vi "首页.vi"() -> ()   [LabVIEW 2016]
uses:
  <vilib>/Utility/miscctls.llb/LVPointTypeDef.ctl
  <vilib>/Utility/sysdir.llb/System Directory Type.ctl
  <vilib>/addons/database/_DB Variant To Data/Database Variant To Data.xnode
  PLC/PLC.lvlib
panel:
  out "大项目框 12":T1(xcontrol)
  out "大项目框 11":T1(xcontrol)
  out "大项目框 10":T1(xcontrol)
  out "大项目框 9":T1(xcontrol)
  out "大项目框 8":T1(xcontrol)
  out "大项目框 7":T1(xcontrol)
  out "大项目框 6":T1(xcontrol)
  out "大项目框 5":T1(xcontrol)
  out "大项目框 4":T1(xcontrol)
  out "大项目框 3":T1(xcontrol)
  out "大项目框 2":T1(xcontrol)
  out "大项目框":T1(xcontrol)
  out "湿度":string="75.5 %"
  out "室温":string="25.8 ℃"
  # "室温:"
  # "湿度:"
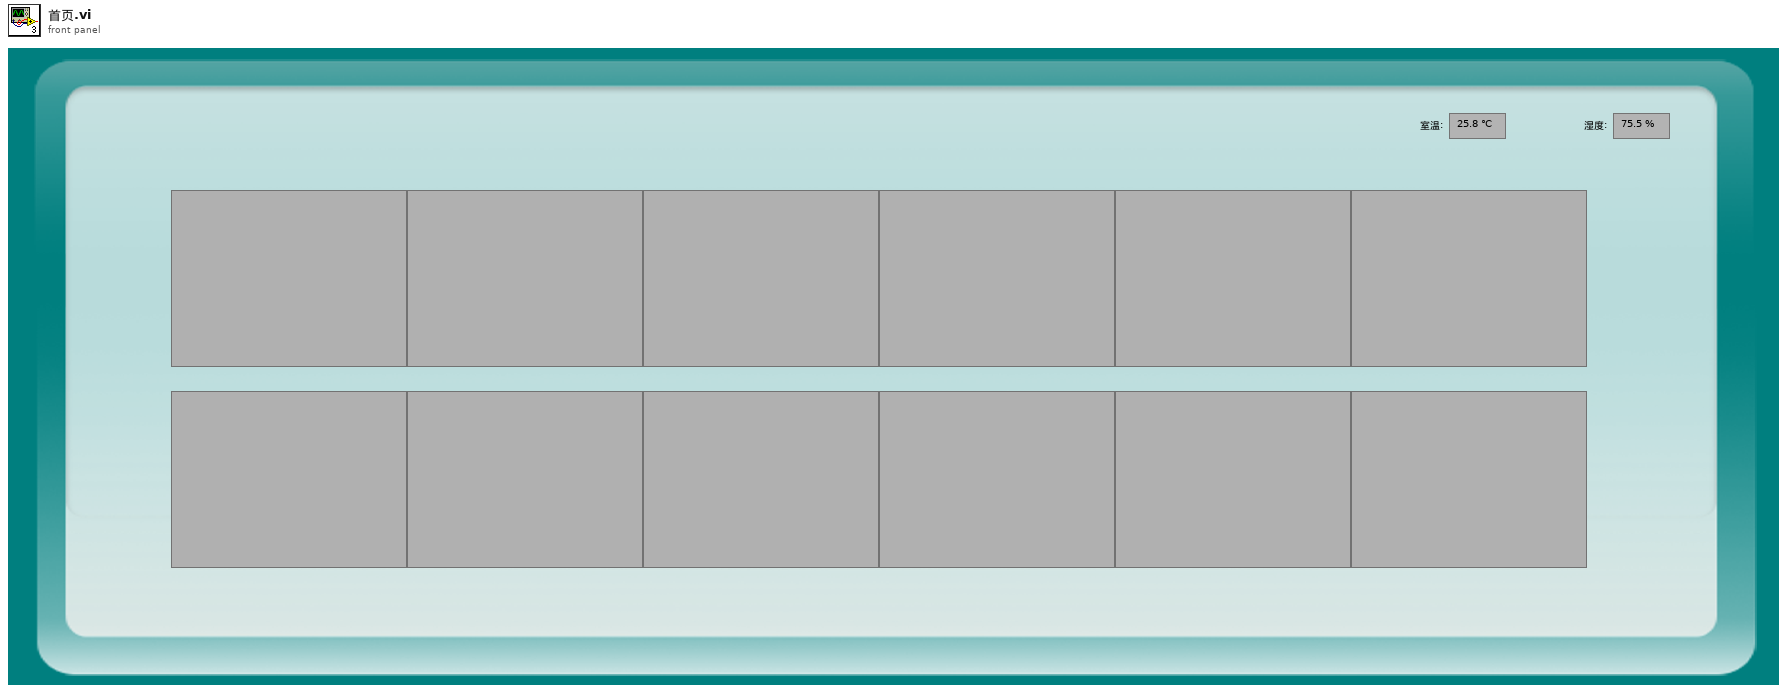
[diagram p1: front panel]
types:
  T1 = cluster{"中文项目名称":string, "英文项目名称":string, "单位":string, "浓度值":string}
  T2 = typedef "LVPointTypeDef.ctl" = cluster{"Horizontal":i16, "Vertical":i16}
  T3 = cluster{"显示参数中文名":string, "显示参数英文名":string, "显示浓度":string, "显示单位":string}[]
  T4 = cluster{"显示参数中文名":string, "显示参数英文名":string, "显示浓度":string, "显示单位":string}
  T5 = typedef "System Directory Type.ctl" = i32
  T6 = cluster{"水温":bool, "pH":bool, "DO":bool, "Cond":bool, "Turb":bool, "氨氮":bool, "总磷":bool, "总氮":bool, "CODMn":bool, "CODCr":bool, "水位":bool, "流速":bool, "瞬时流量":bool, "室温":bool, "湿度":bool}
  T7 = cluster{"AD0":sgl, "AD1":sgl, "AD2":sgl, "AD3":sgl, "AD4":sgl, "AD5":sgl}
  T8 = typedef "LVDateTimeRec.ctl" = cluster{"秒数的小数部分":dbl, "秒":i32, "分":i32, "时":i32, "日":i32, "月":i32, "年":i32, "天数（周）":i32, "天数（年）":i32, "DST":i32}
  T9 = cluster{"时间标识":timestamp, "监测值":sgl, "单位":string}
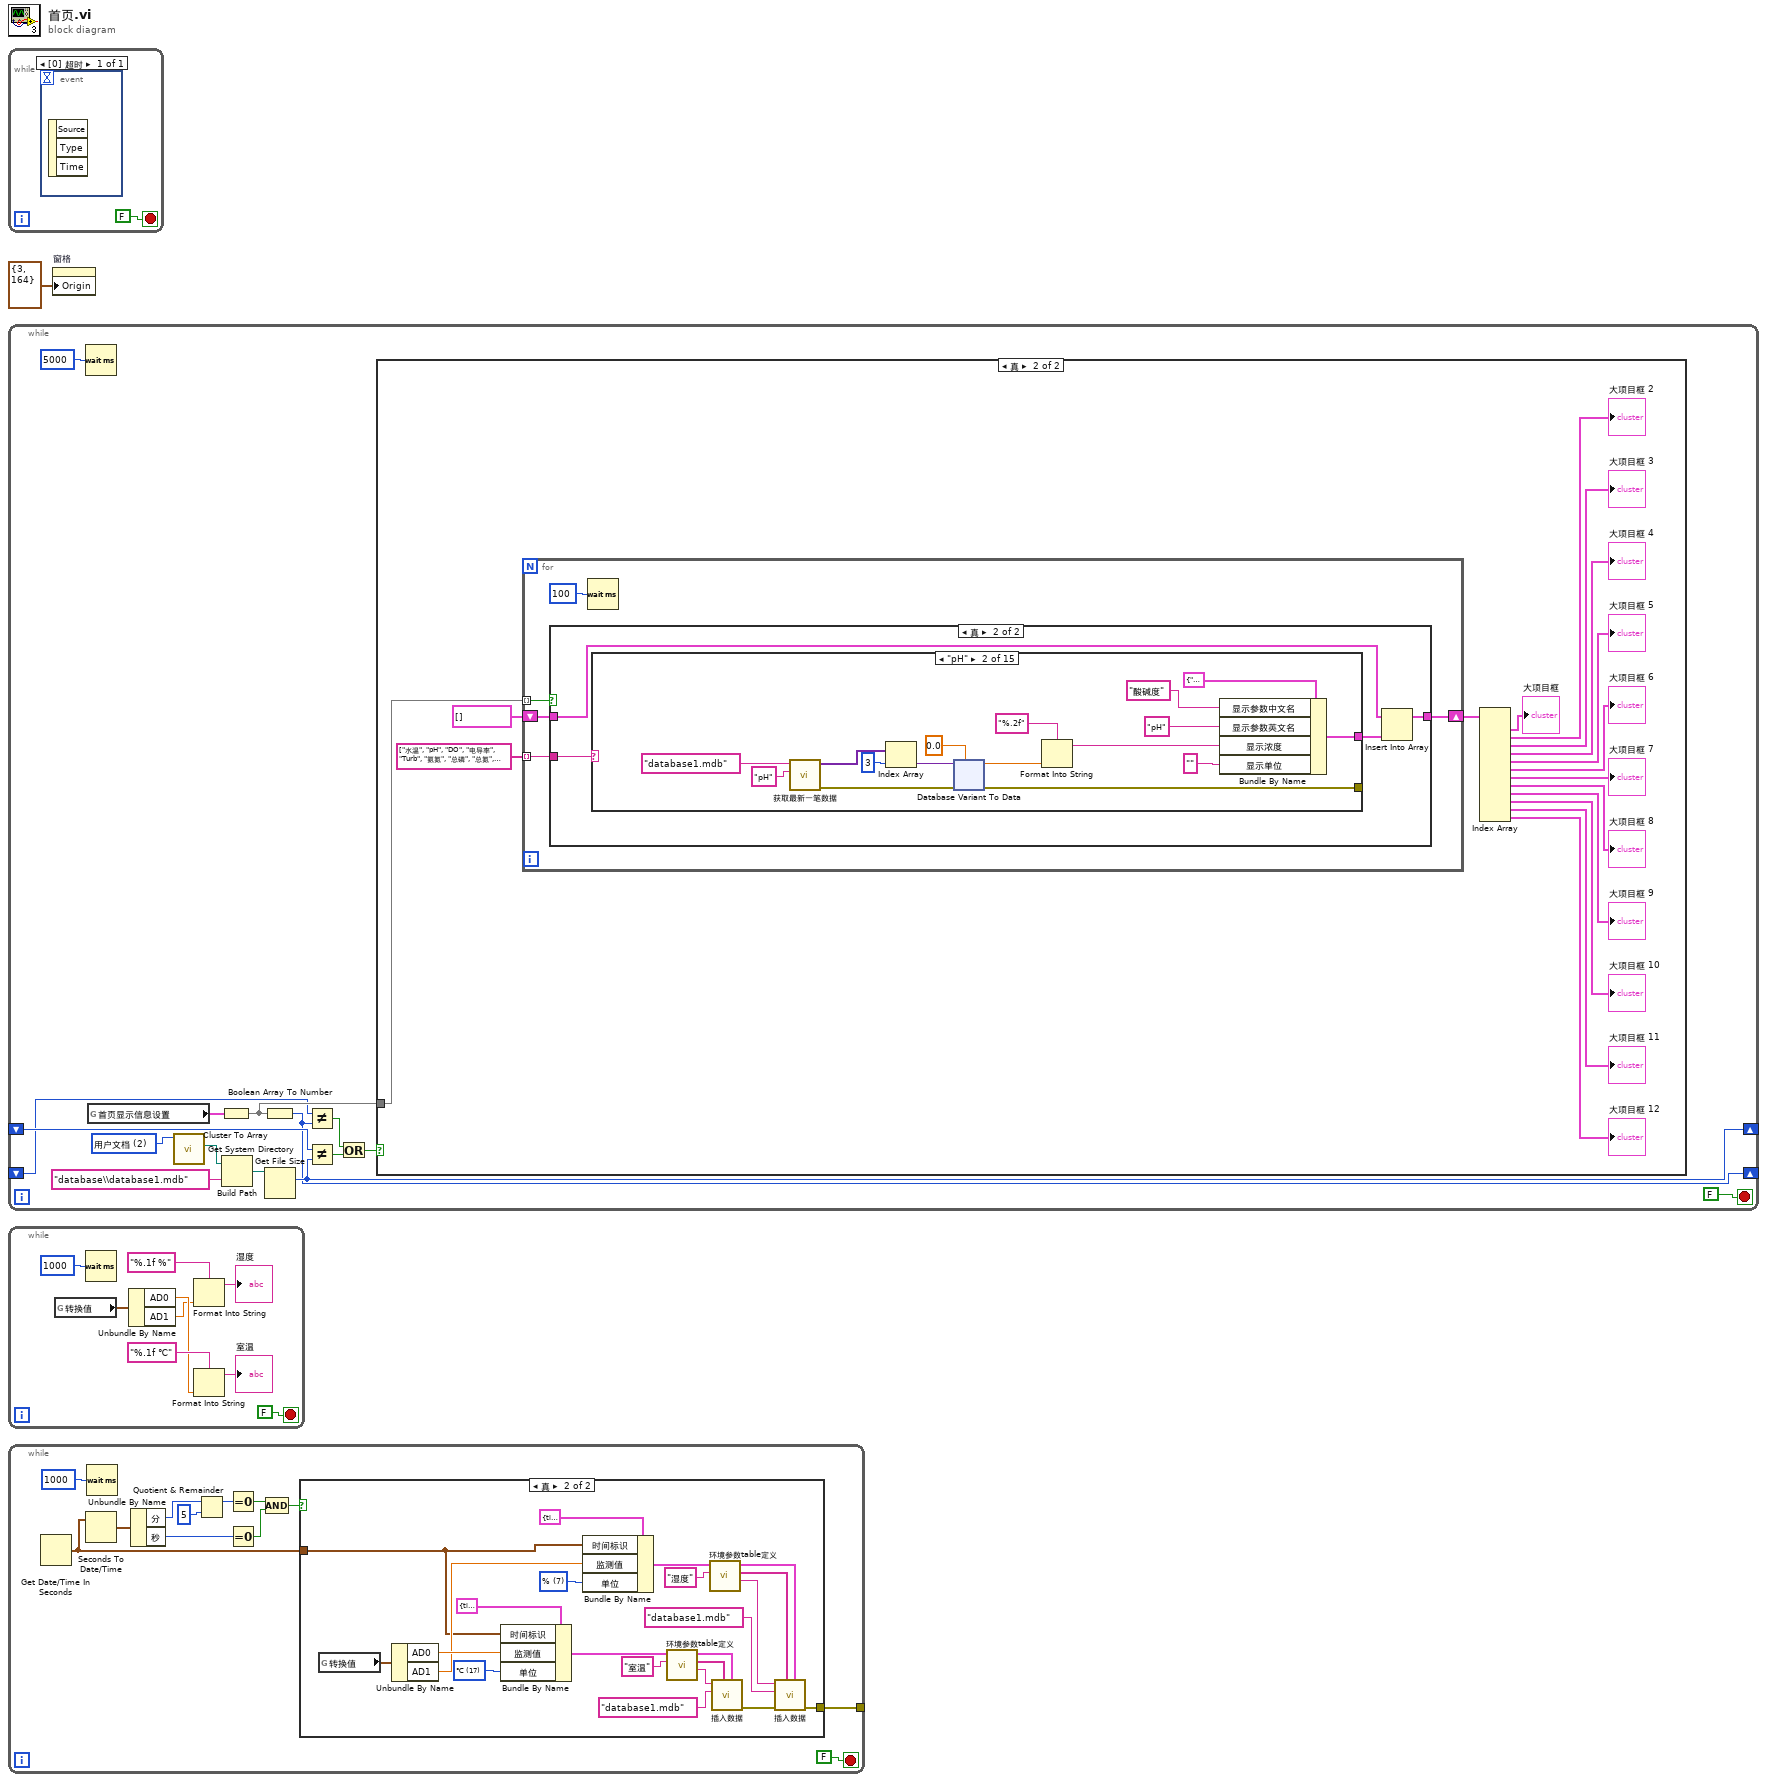
[diagram p0: block diagram]
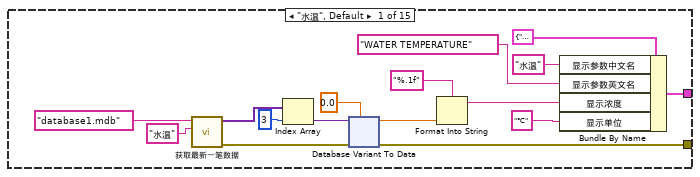
[diagram p5: hidden frame]
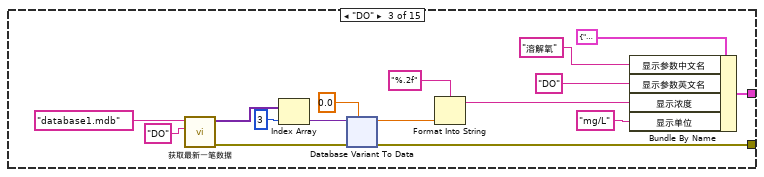
[diagram p6: hidden frame]
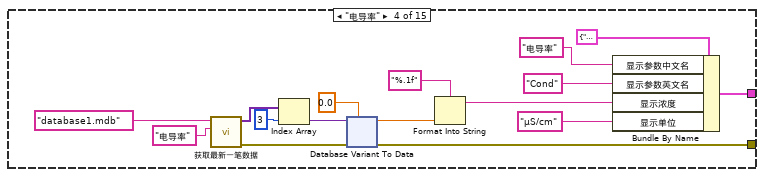
[diagram p7: hidden frame]
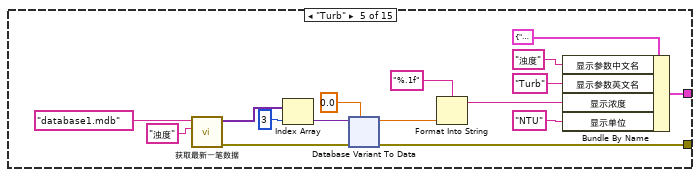
[diagram p8: hidden frame]
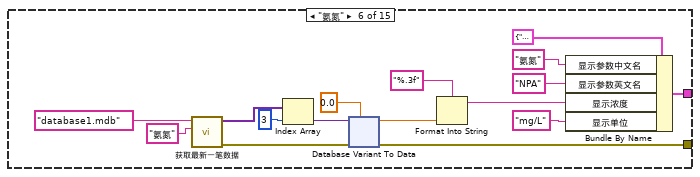
[diagram p9: hidden frame]
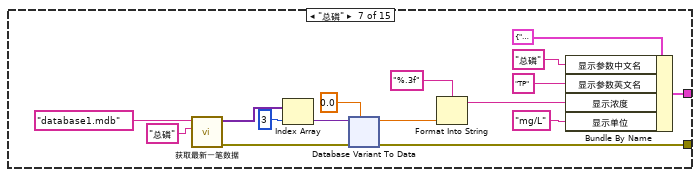
[diagram p10: hidden frame]
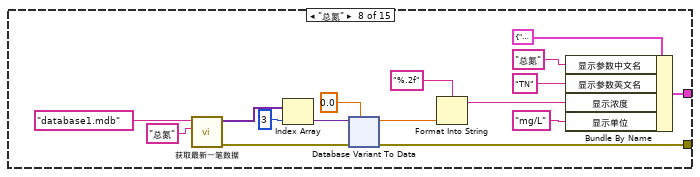
[diagram p11: hidden frame]
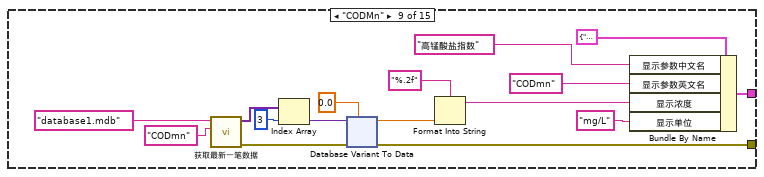
[diagram p12: hidden frame]
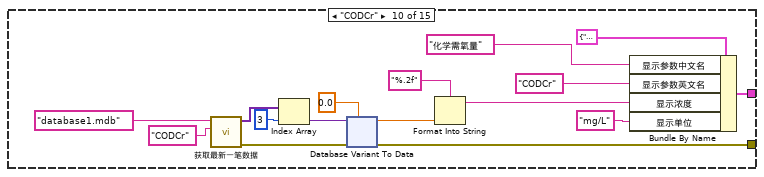
[diagram p13: hidden frame]
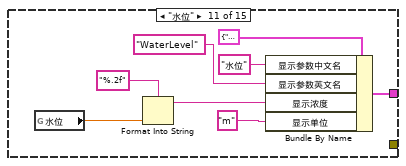
[diagram p14: hidden frame]
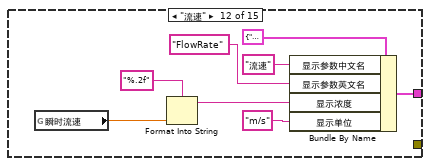
[diagram p15: hidden frame]
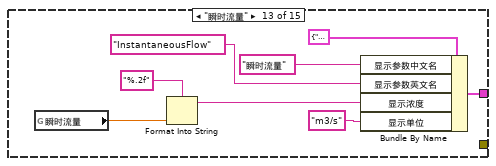
[diagram p16: hidden frame]
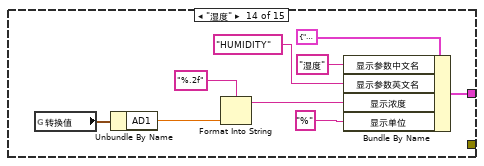
[diagram p17: hidden frame]
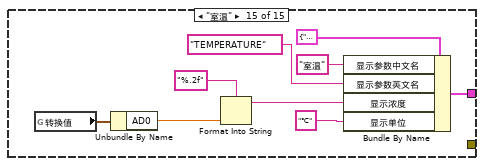
[diagram p18: hidden frame]
diagram:
  n1 = while {
    stop <- FALSE stop-if-true
    n2 = event shown="[0] 超时" {
      selector: _ -> [_]
      dyn-events: _ -> [_]
      timeout: _ -> [_]
      event Timeout {
        n3 = event-data() -> ()  [unwired: 1 in, 3 out]
      }
    }
  }
  n4 = while {
    shift-right: [w9] -> _
    shift-left: _ -> [w10]
    shift-right: [w7] -> _
    shift-left: _ -> [w6]
    stop <- FALSE stop-if-true
    w14 = T5 2 items=["用户目录"=0, "用户桌面"=1, "用户文档"=2, "用户应用程序数据"=3, "用户设置"=4, "用户临时目录"=5, "公共文档"=6, "公共应用程序数据"=7, "公共设置"=8, "公共缓存"=13, "系统核心库"=9, "系统安装库"=10, "应用程序文件"=11, "启动盘根目录"=12] ("system directory type")
    n5 = Wait (ms)(milliseconds to wait=u32 5000 ("等待时间（毫秒）")) -> ()  [unwired: 1 out]
    n6 = global read "系统设置全局变量.vi" "首页显示信息设置"() -> (w15:T6)
    n7 = call <vilib>:"Get System Directory.vi"("system directory type"=w14) -> ("system directory"=w13:path)  [unwired: 10 in]
    n8 = Cluster To Array(cluster=w15) -> (array=w8:bool[])
    n9 = Build Path(base path=w13, name or relative path="database\\database1.mdb" ("名称或相对路径")) -> (appended path=w11:path)
    n10 = Boolean Array To Number(Boolean array=w8) -> (number=w7:u32)
    n11 = Get File Size(file=w11) -> (size (in bytes)=w9:i64)  [unwired: 1 in, 2 out]
    n12 = Not Equal?(x=w6, y=w7) -> (x != y?=w4:bool)
    n13 = Not Equal?(x=w10, y=w9) -> (x != y?=w5:bool)
    n14 = Or(x=w4, y=w5) -> (x .or. y?=w3:bool)
    n15 = case shown="真" w3 {
      tunnel: w8 -> [_ w18]
      frame False {
      }
      frame True {
        n16 = for {
          tunnel: w18 -> [w38] mode=indexing
          tunnel: string[] ["水温", "pH", "DO", "电导率", "Turb", "氨氮", "总磷", "总氮", "CODMn", "CODCr", "水位", "流速", "瞬时流量"] -> [w37] mode=indexing
          shift-right: [w35] -> w31
          shift-left: T3 [] -> [w36]
          n17 = case shown="真" w38 {
            tunnel: w37 -> [_ w43]
            tunnel: w36 -> [w39 w42]
            tunnel: [w39 w41] -> w35
            frame False {
            }
            frame True {
              n18 = case shown="\"pH\"" w43 {
                tunnel: [w44 w103 w151 w199 w247 w295 w343 w391 w439 w487 w527 w535 w540 w552 w561] -> w40
                tunnel: [w45 w92 w140 w188 w236 w284 w332 w380 w428 w476 _ _ _ _ _] -> _
                frame "水温", Default {
                  n19 = call "获取最新一笔数据.vi"("table"="水温", "database"="database1.mdb" ("名称或相对路径")) -> ("error out"=w46:errorcluster, "子数组"=w52:variant[])  [unwired: 8 in]
                  n20 = Index Array(array=w52, index=3 ("索引")) -> (element=w50:variant)
                  n21 = xnode "Database Variant To Data"("database variant"=w50, "error in (no error)"=w46, "type"=0.0) -> ("data"=w47:dbl, "error out"=w45:errorcluster)
                  n22 = Format Into String(format string="%.1f" ("格式字符串"), w47) -> (resulting string=w54:string)  [unwired: 2 in, 1 out]
                  n23 = Bundle By Name(cluster=T4 {"显示参数中文名"="", "显示参数英文名"="", "显示浓度"="", "显示单位"=""} ("元素"), "显示参数中文名"="水温", "显示参数英文名"="WATER TEMPERATURE", "显示浓度"=w54, "显示单位"="℃") -> (w44:T4)
                }
                frame "pH" {
                  n24 = call "获取最新一笔数据.vi"("table"="pH", "database"="database1.mdb" ("名称或相对路径")) -> ("error out"=w93:errorcluster, "子数组"=w99:variant[])  [unwired: 8 in]
                  n25 = Index Array(array=w99, index=3 ("索引")) -> (element=w97:variant)
                  n26 = xnode "Database Variant To Data"("database variant"=w97, "error in (no error)"=w93, "type"=0.0) -> ("data"=w94:dbl, "error out"=w92:errorcluster)
                  n27 = Format Into String(format string="%.2f" ("格式字符串"), w94) -> (resulting string=w101:string)  [unwired: 2 in, 1 out]
                  n28 = Bundle By Name(cluster=T4 {"显示参数中文名"="", "显示参数英文名"="", "显示浓度"="", "显示单位"=""} ("元素"), "显示参数中文名"="酸碱度", "显示参数英文名"="pH", "显示浓度"=w101, "显示单位"="") -> (w103:T4)
                }
                frame "DO" {
                  n29 = call "获取最新一笔数据.vi"("table"="DO", "database"="database1.mdb" ("名称或相对路径")) -> ("error out"=w141:errorcluster, "子数组"=w147:variant[])  [unwired: 8 in]
                  n30 = Index Array(array=w147, index=3 ("索引")) -> (element=w145:variant)
                  n31 = xnode "Database Variant To Data"("database variant"=w145, "error in (no error)"=w141, "type"=0.0) -> ("data"=w142:dbl, "error out"=w140:errorcluster)
                  n32 = Format Into String(format string="%.2f" ("格式字符串"), w142) -> (resulting string=w149:string)  [unwired: 2 in, 1 out]
                  n33 = Bundle By Name(cluster=T4 {"显示参数中文名"="", "显示参数英文名"="", "显示浓度"="", "显示单位"=""} ("元素"), "显示参数中文名"="溶解氧", "显示参数英文名"="DO", "显示浓度"=w149, "显示单位"="mg/L") -> (w151:T4)
                }
                frame "电导率" {
                  n34 = call "获取最新一笔数据.vi"("table"="电导率", "database"="database1.mdb" ("名称或相对路径")) -> ("error out"=w189:errorcluster, "子数组"=w195:variant[])  [unwired: 8 in]
                  n35 = Index Array(array=w195, index=3 ("索引")) -> (element=w193:variant)
                  n36 = xnode "Database Variant To Data"("database variant"=w193, "error in (no error)"=w189, "type"=0.0) -> ("data"=w190:dbl, "error out"=w188:errorcluster)
                  n37 = Format Into String(format string="%.1f" ("格式字符串"), w190) -> (resulting string=w197:string)  [unwired: 2 in, 1 out]
                  n38 = Bundle By Name(cluster=T4 {"显示参数中文名"="", "显示参数英文名"="", "显示浓度"="", "显示单位"=""} ("元素"), "显示参数中文名"="电导率", "显示参数英文名"="Cond", "显示浓度"=w197, "显示单位"="μS/cm") -> (w199:T4)
                }
                frame "Turb" {
                  n39 = call "获取最新一笔数据.vi"("table"="浊度", "database"="database1.mdb" ("名称或相对路径")) -> ("error out"=w237:errorcluster, "子数组"=w243:variant[])  [unwired: 8 in]
                  n40 = Index Array(array=w243, index=3 ("索引")) -> (element=w241:variant)
                  n41 = xnode "Database Variant To Data"("database variant"=w241, "error in (no error)"=w237, "type"=0.0) -> ("data"=w238:dbl, "error out"=w236:errorcluster)
                  n42 = Format Into String(format string="%.1f" ("格式字符串"), w238) -> (resulting string=w245:string)  [unwired: 2 in, 1 out]
                  n43 = Bundle By Name(cluster=T4 {"显示参数中文名"="", "显示参数英文名"="", "显示浓度"="", "显示单位"=""} ("元素"), "显示参数中文名"="浊度", "显示参数英文名"="Turb", "显示浓度"=w245, "显示单位"="NTU") -> (w247:T4)
                }
                frame "氨氮" {
                  n44 = call "获取最新一笔数据.vi"("table"="氨氮", "database"="database1.mdb" ("名称或相对路径")) -> ("error out"=w285:errorcluster, "子数组"=w291:variant[])  [unwired: 8 in]
                  n45 = Index Array(array=w291, index=3 ("索引")) -> (element=w289:variant)
                  n46 = xnode "Database Variant To Data"("database variant"=w289, "error in (no error)"=w285, "type"=0.0) -> ("data"=w286:dbl, "error out"=w284:errorcluster)
                  n47 = Format Into String(format string="%.3f" ("格式字符串"), w286) -> (resulting string=w293:string)  [unwired: 2 in, 1 out]
                  n48 = Bundle By Name(cluster=T4 {"显示参数中文名"="", "显示参数英文名"="", "显示浓度"="", "显示单位"=""} ("元素"), "显示参数中文名"="氨氮", "显示参数英文名"="NPA", "显示浓度"=w293, "显示单位"="mg/L") -> (w295:T4)
                }
                frame "总磷" {
                  n49 = call "获取最新一笔数据.vi"("table"="总磷", "database"="database1.mdb" ("名称或相对路径")) -> ("error out"=w333:errorcluster, "子数组"=w339:variant[])  [unwired: 8 in]
                  n50 = Index Array(array=w339, index=3 ("索引")) -> (element=w337:variant)
                  n51 = xnode "Database Variant To Data"("database variant"=w337, "error in (no error)"=w333, "type"=0.0) -> ("data"=w334:dbl, "error out"=w332:errorcluster)
                  n52 = Format Into String(format string="%.3f" ("格式字符串"), w334) -> (resulting string=w341:string)  [unwired: 2 in, 1 out]
                  n53 = Bundle By Name(cluster=T4 {"显示参数中文名"="", "显示参数英文名"="", "显示浓度"="", "显示单位"=""} ("元素"), "显示参数中文名"="总磷", "显示参数英文名"="TP", "显示浓度"=w341, "显示单位"="mg/L") -> (w343:T4)
                }
                frame "总氮" {
                  n54 = call "获取最新一笔数据.vi"("table"="总氮", "database"="database1.mdb" ("名称或相对路径")) -> ("error out"=w381:errorcluster, "子数组"=w387:variant[])  [unwired: 8 in]
                  n55 = Index Array(array=w387, index=3 ("索引")) -> (element=w385:variant)
                  n56 = xnode "Database Variant To Data"("database variant"=w385, "error in (no error)"=w381, "type"=0.0) -> ("data"=w382:dbl, "error out"=w380:errorcluster)
                  n57 = Format Into String(format string="%.2f" ("格式字符串"), w382) -> (resulting string=w389:string)  [unwired: 2 in, 1 out]
                  n58 = Bundle By Name(cluster=T4 {"显示参数中文名"="", "显示参数英文名"="", "显示浓度"="", "显示单位"=""} ("元素"), "显示参数中文名"="总氮", "显示参数英文名"="TN", "显示浓度"=w389, "显示单位"="mg/L") -> (w391:T4)
                }
                frame "CODMn" {
                  n59 = call "获取最新一笔数据.vi"("table"="CODmn", "database"="database1.mdb" ("名称或相对路径")) -> ("error out"=w429:errorcluster, "子数组"=w435:variant[])  [unwired: 8 in]
                  n60 = Index Array(array=w435, index=3 ("索引")) -> (element=w433:variant)
                  n61 = xnode "Database Variant To Data"("database variant"=w433, "error in (no error)"=w429, "type"=0.0) -> ("data"=w430:dbl, "error out"=w428:errorcluster)
                  n62 = Format Into String(format string="%.2f" ("格式字符串"), w430) -> (resulting string=w437:string)  [unwired: 2 in, 1 out]
                  n63 = Bundle By Name(cluster=T4 {"显示参数中文名"="", "显示参数英文名"="", "显示浓度"="", "显示单位"=""} ("元素"), "显示参数中文名"="高锰酸盐指数", "显示参数英文名"="CODmn", "显示浓度"=w437, "显示单位"="mg/L") -> (w439:T4)
                }
                frame "CODCr" {
                  n64 = call "获取最新一笔数据.vi"("table"="CODCr", "database"="database1.mdb" ("名称或相对路径")) -> ("error out"=w477:errorcluster, "子数组"=w483:variant[])  [unwired: 8 in]
                  n65 = Index Array(array=w483, index=3 ("索引")) -> (element=w481:variant)
                  n66 = xnode "Database Variant To Data"("database variant"=w481, "error in (no error)"=w477, "type"=0.0) -> ("data"=w478:dbl, "error out"=w476:errorcluster)
                  n67 = Format Into String(format string="%.2f" ("格式字符串"), w478) -> (resulting string=w485:string)  [unwired: 2 in, 1 out]
                  n68 = Bundle By Name(cluster=T4 {"显示参数中文名"="", "显示参数英文名"="", "显示浓度"="", "显示单位"=""} ("元素"), "显示参数中文名"="化学需氧量", "显示参数英文名"="CODCr", "显示浓度"=w485, "显示单位"="mg/L") -> (w487:T4)
                }
                frame "水位" {
                  n69 = global read "流量计全局变量.vi" "水位"() -> (w524:dbl)
                  n70 = Format Into String(format string="%.2f" ("格式字符串"), w524) -> (resulting string=w525:string)  [unwired: 2 in, 1 out]
                  n71 = Bundle By Name(cluster=T4 {"显示参数中文名"="", "显示参数英文名"="", "显示浓度"="", "显示单位"=""} ("元素"), "显示参数中文名"="水位", "显示参数英文名"="WaterLevel", "显示浓度"=w525, "显示单位"="m") -> (w527:T4)
                }
                frame "流速" {
                  n72 = global read "流量计全局变量.vi" "瞬时流速"() -> (w532:dbl)
                  n73 = Format Into String(format string="%.2f" ("格式字符串"), w532) -> (resulting string=w533:string)  [unwired: 2 in, 1 out]
                  n74 = Bundle By Name(cluster=T4 {"显示参数中文名"="", "显示参数英文名"="", "显示浓度"="", "显示单位"=""} ("元素"), "显示参数中文名"="流速", "显示参数英文名"="FlowRate", "显示浓度"=w533, "显示单位"="m/s") -> (w535:T4)
                }
                frame "瞬时流量" {
                  n75 = global read "流量计全局变量.vi" "瞬时流量"() -> (w541:dbl)
                  n76 = Format Into String(format string="%.2f" ("格式字符串"), w541) -> (resulting string=w542:string)  [unwired: 2 in, 1 out]
                  n77 = Bundle By Name(cluster=T4 {"显示参数中文名"="", "显示参数英文名"="", "显示浓度"="", "显示单位"=""} ("元素"), "显示参数中文名"="瞬时流量", "显示参数英文名"="InstantaneousFlow", "显示浓度"=w542, "显示单位"="m3/s") -> (w540:T4)
                }
                frame "湿度" {
                  n78 = global read "采配水全局变量.vi" "转换值"() -> (w549:T7)
                  n79 = Unbundle By Name(w549) -> ("AD1"=w551:sgl)
                  n80 = Format Into String(format string="%.2f" ("格式字符串"), w551) -> (resulting string=w548:string)  [unwired: 2 in, 1 out]
                  n81 = Bundle By Name(cluster=T4 {"显示参数中文名"="", "显示参数英文名"="", "显示浓度"="", "显示单位"=""} ("元素"), "显示参数中文名"="湿度", "显示参数英文名"="HUMIDITY", "显示浓度"=w548, "显示单位"="%") -> (w552:T4)
                }
                frame "室温" {
                  n82 = global read "采配水全局变量.vi" "转换值"() -> (w558:T7)
                  n83 = Unbundle By Name(w558) -> ("AD0"=w560:sgl)
                  n84 = Format Into String(format string="%.2f" ("格式字符串"), w560) -> (resulting string=w557:string)  [unwired: 2 in, 1 out]
                  n85 = Bundle By Name(cluster=T4 {"显示参数中文名"="", "显示参数英文名"="", "显示浓度"="", "显示单位"=""} ("元素"), "显示参数中文名"="室温", "显示参数英文名"="TEMPERATURE", "显示浓度"=w557, "显示单位"="℃") -> (w561:T4)
                }
              }
              n86 = Insert Into Array(array=w42, new element=w40) -> (w41:T3)  [unwired: 1 in]
            }
          }
          n87 = Wait (ms)(milliseconds to wait=u32 100 ("等待时间（毫秒）")) -> ()  [unwired: 1 out]
        }
        n88 = Index Array(array=w31) -> (element #1=→"大项目框":T4, element #2=→"大项目框 2":T4, element #3=→"大项目框 3":T4, element #4=→"大项目框 4":T4, element #5=→"大项目框 5":T4, element #6=→"大项目框 6":T4, element #7=→"大项目框 7":T4, element #8=→"大项目框 8":T4, element #9=→"大项目框 9":T4, element #10=→"大项目框 10":T4, element #11=→"大项目框 11":T4, element #12=→"大项目框 12":T4)  [unwired: 12 in]
      }
    }
  }
  n89 = while {
    stop <- FALSE stop-if-true
    n90 = global read "采配水全局变量.vi" "转换值"() -> (w572:T7)
    n91 = Wait (ms)(milliseconds to wait=u32 1000 ("等待时间（毫秒）")) -> ()  [unwired: 1 out]
    n92 = Unbundle By Name(w572) -> ("AD0"=w567:sgl, "AD1"=w566:sgl)
    n93 = Format Into String(format string="%.1f %" ("格式字符串"), w566) -> (resulting string=→"湿度":string)  [unwired: 2 in, 1 out]
    n94 = Format Into String(format string="%.1f ℃" ("格式字符串"), w567) -> (resulting string=→"室温":string)  [unwired: 2 in, 1 out]
  }
  n95 = while {
    tunnel: [w585] -> _
    stop <- FALSE stop-if-true
    n96 = Get Date/Time In Seconds() -> (seconds since 1Jan1904=w584:timestamp)
    n97 = Seconds To Date/Time(time stamp (now)=w584) -> (date time rec=w583:T8)  [unwired: 1 in]
    n98 = Wait (ms)(milliseconds to wait=u32 1000 ("等待时间（毫秒）")) -> ()  [unwired: 1 out]
    n99 = Unbundle By Name(w583) -> ("分"=w582:i32, "秒"=w580:i32)
    n100 = Quotient & Remainder(x=w582, y=5) -> (x-y*floor(x/y)=w579:i32)  [unwired: 1 out]
    n101 = Equal To 0?(x=w579) -> (x = 0?=w578:bool)
    n102 = Equal To 0?(x=w580) -> (x = 0?=w577:bool)
    n103 = Compound Arithmetic op=AND ("复合运算")(w578, w577) -> (w576:bool)
    n104 = case shown="真" w576 {
      tunnel: [_ w600] -> w585
      tunnel: w584 -> [_ w588]
      frame False {
      }
      frame True {
        w593 = u16 7 items=["ug/L", "mg/L", "ppm", "mg/m3", "cm", "ppb", "ug/m3", "%", "nmol/mol", "umol/mol", "MPN/L", "MPN/100ml", "ng/m3", "NTU", "无量纲", "ms/cm", "us/cm", "℃", "V"] ("单位")
        w597 = u16 17 items=["ug/L", "mg/L", "ppm", "mg/m3", "cm", "ppb", "ug/m3", "%", "nmol/mol", "umol/mol", "MPN/L", "MPN/100ml", "ng/m3", "NTU", "无量纲", "ms/cm", "us/cm", "℃", "V"] ("单位")
        n105 = global read "采配水全局变量.vi" "转换值"() -> (w608:T7)
        n106 = Unbundle By Name(w608) -> ("AD0"=w596:sgl, "AD1"=w594:sgl)
        n107 = Bundle By Name(cluster=cluster{"时间标识":timestamp, "监测值":sgl, "单位":u16} {"时间标识"=timestamp(0 s since 1904-01-01), "监测值"=0.0, "单位"=0} ("data"), "时间标识"=w588, "监测值"=w596, "单位"=w597) -> (w598:cluster{"时间标识":timestamp, "监测值":sgl, "单位":u16})
        n108 = Bundle By Name(cluster=cluster{"时间标识":timestamp, "监测值":sgl, "单位":u16} {"时间标识"=timestamp(0 s since 1904-01-01), "监测值"=0.0, "单位"=0} ("data"), "时间标识"=w588, "监测值"=w594, "单位"=w593) -> (w592:cluster{"时间标识":timestamp, "监测值":sgl, "单位":u16})
        n109 = call "环境参数table定义.vi"("table 输入"="室温", "data"=w598) -> ("table 输出"=w607:string, "columns"=w606:string[], "data输出"=w605:T9)  [unwired: 7 in]
        n110 = call "环境参数table定义.vi"("table 输入"="湿度", "data"=w592) -> ("table 输出"=w602:string, "columns"=w603:string[], "data输出"=w604:T9)  [unwired: 7 in]
        n111 = call "插入数据.vi"("data"=w605, "columns"=w606, "database"="database1.mdb" ("table 输入"), "table"=w607) -> ("error out"=w601:errorcluster)  [unwired: 7 in]
        n112 = call "插入数据.vi"("data"=w604, "columns"=w603, "error in (no error)"=w601, "database"="database1.mdb" ("table 输入"), "table"=w602) -> ("error out"=w600:errorcluster)  [unwired: 6 in]
      }
    }
  }
  n113 = property on="窗格" class="Pane"("Origin"=T2 {"Horizontal"=3, "Vertical"=164} ("原点")) -> ()  [unwired: 2 in, 2 out]
